vi "File_Create Menu Element.vi"(7 "Run Data":T1={"Target Folder"=path "", "Menu Folder"=path "", "Active Folder"=path "", "Config"={"Main"={"Menu Folder"="", "Re-Create Menu Folder?"=FALSE, "Allow mnu replace?"=FALSE}, "File Filter"={"Exclude Prefixes"=[], "Ignore Names"=[], "Include Extensions"=[], "Exclude Postfixes"=[]}, "Folder Filter"={"Exclude Prefixes"=[], "Ignore Names"=[]}, "File Name Edit"={"Pre Split String"="", "Post Split String"=""}, "Folder Name Edit"={"Pre Split String"="", "Post Split String"="", "Deletion Strings"=[]}, "Folder Icon Map"={}, "Default Palette Data"={"Display Name Override"="", "View Format"=2, "Palette Width"=0, "Help Tag"="", "Help File Path"=path "", "Palette Description"=""}, "Default File Data"={"Display Name Override"="", "Place VI Contents?"=FALSE}, "Palette Override map"={}, "File Override map"={}}} {"Config"."Default Palette Data"."View Format" items=["Icons", "Text", "Icons and Text"]}, 8 "error in (no error)":errorcluster, 11 "Valid File Paths":path[](array[path])) -> (0 "error out":errorcluster, 3 "Array":T12[](array[typedef]))   [LabVIEW 2019, in "AutoMenuCreator.lvlib"]
uses:
  AutoMenuCreator.lvlib
  <vilib>/Palette API/Palette Menu/Public Type Define/Item.ctl
  Ctl/Ctl_Run Data.ctl
  Ctl/Ctl_Config.ctl
  Ctl/Ctl_Config_Main.ctl
  Ctl/Ctl_Config_File Filter.ctl
  Ctl/Ctl_Config_Folder Filter.ctl
  Ctl/Ctl_Config_File Name Edit.ctl
  Ctl/Ctl_Config_Folder Name Edit.ctl
  Ctl/Ctl_Config_Folder Icon Map.ctl
  <vilib>/Palette API/Palette Menu/Palette Menu.lvlib
  <vilib>/Palette API/Palette Menu/Public Type Define/View Format.ctl
  Ctl/Ctl_Config_Palette Data.ctl
  Ctl/Ctl_Config_File Data.ctl
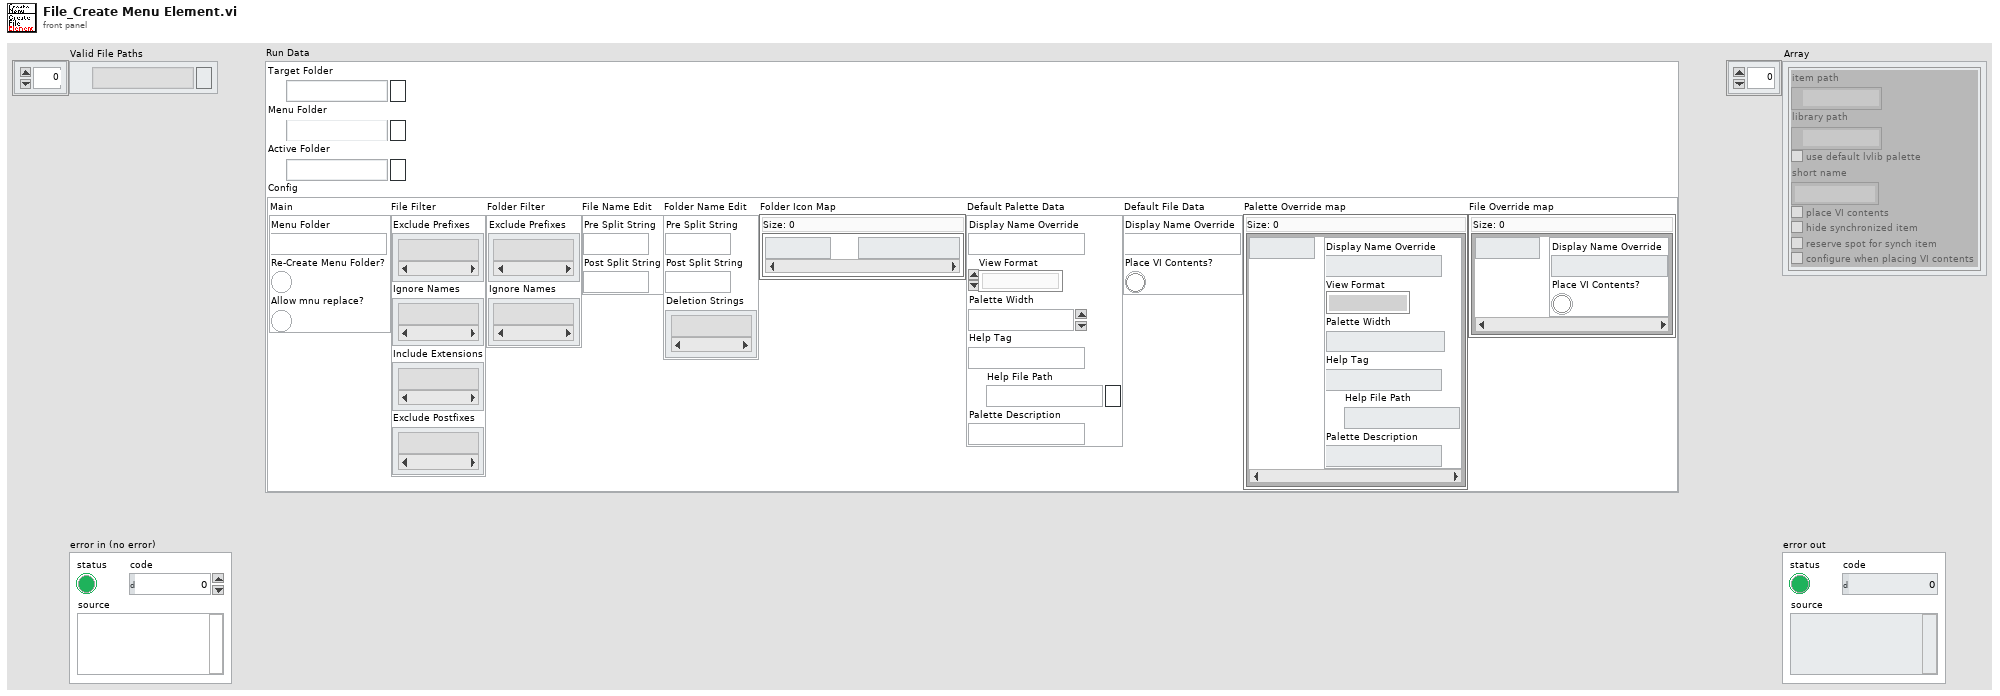
[diagram p1: front panel]
types:
  T1 = typedef "AutoMenuCreator.lvlib/Ctl_Run Data.ctl" = cluster{"Target Folder":path, "Menu Folder":path, "Active Folder":path, "Config":T2}
  T2 = typedef "AutoMenuCreator.lvlib/Ctl_Config.ctl" = cluster{"Main":T3, "File Filter":T4, "Folder Filter":T5, "File Name Edit":T6, "Folder Name Edit":T7, "Folder Icon Map":T8, "Default Palette Data":T9, "Default File Data":T11, "Palette Override map":map{string, T9}, "File Override map":map{string, T11}}
  T3 = typedef "AutoMenuCreator.lvlib/Ctl_Config_Main.ctl" = cluster{"Menu Folder":string, "Re-Create Menu Folder?":bool, "Allow mnu replace?":bool}
  T4 = typedef "AutoMenuCreator.lvlib/Ctl_Config_File Filter.ctl" = cluster{"Exclude Prefixes":string[], "Ignore Names":string[], "Include Extensions":string[], "Exclude Postfixes":string[]}
  T5 = typedef "AutoMenuCreator.lvlib/Ctl_Config_Folder Filter.ctl" = cluster{"Exclude Prefixes":string[], "Ignore Names":string[]}
  T6 = typedef "AutoMenuCreator.lvlib/Ctl_Config_File Name Edit.ctl" = cluster{"Pre Split String":string, "Post Split String":string}
  T7 = typedef "AutoMenuCreator.lvlib/Ctl_Config_Folder Name Edit.ctl" = cluster{"Pre Split String":string, "Post Split String":string, "Deletion Strings":string[]}
  T8 = typedef "AutoMenuCreator.lvlib/Ctl_Config_Folder Icon Map.ctl" = map{string, path}
  T9 = typedef "AutoMenuCreator.lvlib/Ctl_Config_Palette Data.ctl" = cluster{"Display Name Override":string, "View Format":T10, "Palette Width":i16, "Help Tag":string, "Help File Path":path, "Palette Description":string}
  T10 = typedef "Palette Menu.lvlib/View Format.ctl" = u16
  T11 = typedef "AutoMenuCreator.lvlib/Ctl_Config_File Data.ctl" = cluster{"Display Name Override":string, "Place VI Contents?":bool}
  T12 = typedef "Palette Menu.lvlib/Item.ctl" = cluster{"item path":path, "library path":path, "use default lvlib palette":bool, "short name":string, "place VI contents":bool, "hide synchronized item":bool, "reserve spot for synch item":bool, "configure when placing VI contents":bool}
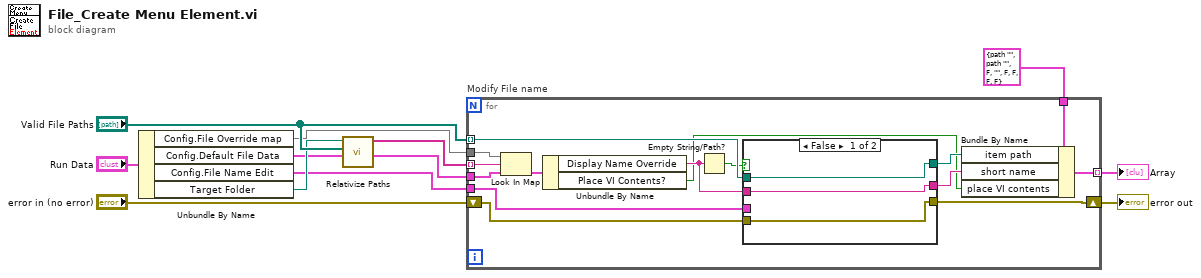
[diagram p0: block diagram]
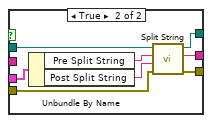
[diagram p2: hidden frame]
diagram:
  n1 = Unbundle By Name("Run Data") -> ("Config.File Override map"=w2:map{string, T11}, "Config.Default File Data"=w1:T11, "Config.File Name Edit"=w4:T6, "Target Folder"=w5:path)
  n2 = call "Relativize Paths.vi"("Valid File Paths"="Valid File Paths", "Target Folder"=w5) -> ("Array"=w7:string[])  [unwired: 9 in]
  n3 = for "Modify File name" {
    tunnel: T12 {"item path"=path "", "library path"=path "", "use default lvlib palette"=FALSE, "short name"="", "place VI contents"=FALSE, "hide synchronized item"=FALSE, "reserve spot for synch item"=FALSE, "configure when placing VI contents"=FALSE} ("items") -> [w26]
    tunnel: "Valid File Paths" -> [w23] mode=indexing
    tunnel: [w25] -> w9 mode=indexing
    shift-right: [w20] -> w11
    shift-left: "error in (no error)" -> [w21]
    tunnel: w4 -> [w19]
    tunnel: w7 -> [w18] mode=indexing
    tunnel: w2 -> [w17]
    tunnel: w1 -> [w16]
    n4 = Look In Map(map=w17, key=w18, default value=w16) -> (value=w15:T11)  [unwired: 1 out]
    n5 = Unbundle By Name(w15) -> ("Display Name Override"=w13:string, "Place VI Contents?"=w12:bool)
    n6 = Empty String/Path?(string/path=w13) -> (empty?=w14:bool)
    n7 = case shown="False" w14 {
      tunnel: [w28 w37] -> w24
      tunnel: w23 -> [w28 w36]
      tunnel: [w29 w35] -> w22
      tunnel: w21 -> [w27 w34]
      tunnel: [w27 w33] -> w20
      tunnel: w19 -> [_ w32]
      tunnel: w13 -> [w29 _]
      frame False {
      }
      frame True {
        n8 = Unbundle By Name(w32) -> ("Pre Split String"=w31:string, "Post Split String"=w30:string)
        n9 = call "Split String.vi"("error in (no error)"=w34, "Post Split"=w30, "Pre Split"=w31, "Path in"=w36) -> ("error out"=w33:errorcluster, "Formatted name"=w35:string, "Dup Path out"=w37:path)  [unwired: 5 in]
      }
    }
    n10 = Bundle By Name(cluster=w26, "item path"=w24, "short name"=w22, "place VI contents"=w12) -> (w25:T12)
  }
  "error out" <- w11
  "Array" <- w9
